vi "Add Result.vi"(8 "error in (no error)":errorcluster, 10 "Step":refnum<class "Step.lvclass">, 11 "Sequence in":refnum<class "Sequence.lvclass">) -> (0 "error out":errorcluster, 3 "Sequence out":refnum<class "Sequence.lvclass">)   [LabVIEW 2015, in "Sequence.lvclass"]
uses:
  Sequence.lvclass
  Step/Execution/Step.lvclass
  Sequence.lvclass/Sequence.ctl
  Result/Result.lvclass
  Results List/Results List.lvclass
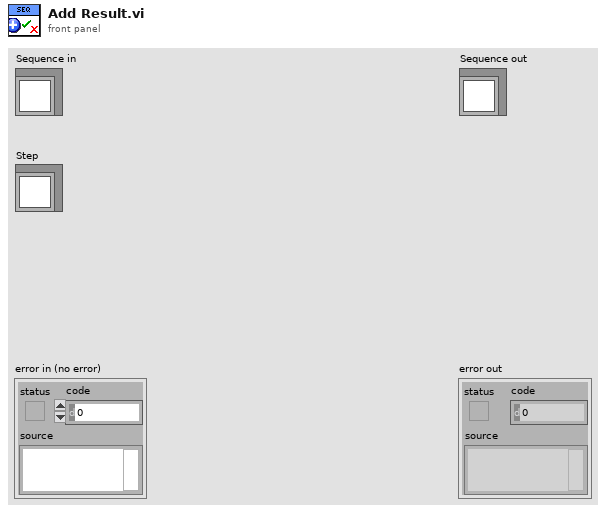
[diagram p1: front panel]
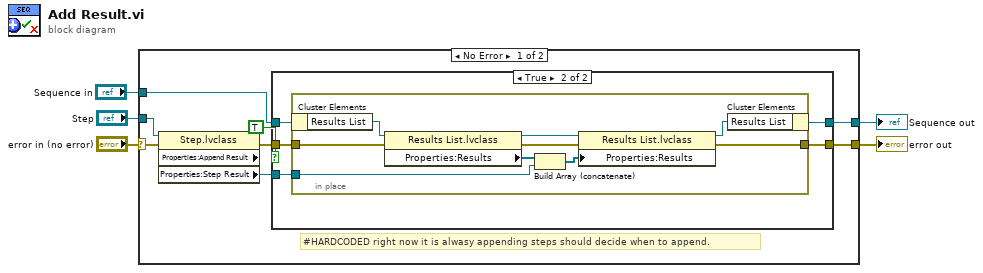
[diagram p0: block diagram]
diagram:
  n1 = case shown="No Error" "error in (no error)" {
    selector: "error in (no error)" -> [w9 w31]
    tunnel: [w10 w31] -> w4
    tunnel: [w7 w30] -> w2
    tunnel: "Sequence in" -> [w8 w30]
    tunnel: "Step" -> [w13 _]
    frame No Error {
      # "#HARDCODED right now it is alwasy appending steps should decide when to append."
      n2 = property class="Step.lvclass" props=["Properties:Append Result", "Properties:Step Result"](reference=w13, error in=w9) -> (error out=w11:errorcluster, "Properties:Step Result"=w12:refnum<class "Result.lvclass">)  [unwired: 2 out]
      n3 = case shown="True" TRUE {
        tunnel: w12 -> [_ w20]
        tunnel: w11 -> [w14 w19]
        tunnel: [w14 w18] -> w10
        tunnel: w8 -> [w15 w17]
        tunnel: [w15 w16] -> w7
        frame False {
        }
        frame True {
          n4 = in-place {
            in-place-border: w20 -> [w27]
            in-place-border: w19 -> [w25]
            in-place-border: [w23] -> w18
            n5 = in-place-cluster #1(w17) -> ("Results List"=w22:refnum<class "Results List.lvclass">)
            n6 = property class="Results List.lvclass"(reference=w22, error in=w25) -> (reference out=w29:refnum<class "Results List.lvclass">, error out=w24:errorcluster, "Properties:Results"=w28:refnum<class "Result.lvclass">[])
            n7 = Build Array (concatenate)(w28, w27) -> (w26:refnum<class "Result.lvclass">[])
            n8 = property class="Results List.lvclass"(reference=w29, error in=w24, "Properties:Results"=w26) -> (reference out=w21:refnum<class "Results List.lvclass">, error out=w23:errorcluster)
            n9 = in-place-cluster #1("Results List"=w21) -> (w16:refnum<class "Sequence.lvclass">)
          }
        }
      }
    }
    frame Error {
    }
  }
  "error out" <- w4
  "Sequence out" <- w2
